vi "Untitled 3.vi"() -> ()   [LabVIEW 2020]
panel:
  out "AREA DEL TRIANGULO":dbl
  in  "ALTURA DE TRIANGULO":dbl
  in  "BASE DEL TRIANGULO":dbl
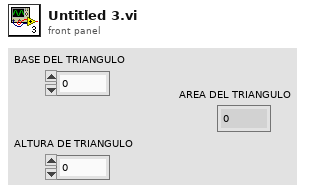
[diagram p1: front panel]
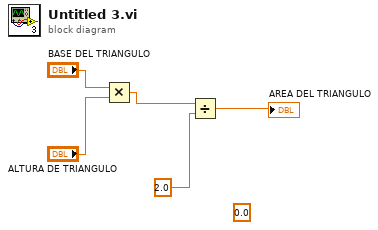
[diagram p0: block diagram]
diagram:
  (unwired) 0.0
  n1 = Multiply(x="BASE DEL TRIANGULO", y="ALTURA DE TRIANGULO") -> (x*y=w3:dbl)
  n2 = Divide(x=w3, y=2.0) -> (x/y=→"AREA DEL TRIANGULO":dbl)
